vi "Set VI Icon Demo.vi"() -> ()   [LabVIEW 2013]
panel:
  out "Icon File":path
  in  "停止":bool
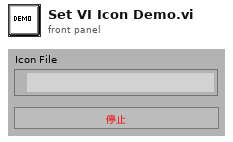
[diagram p1: front panel]
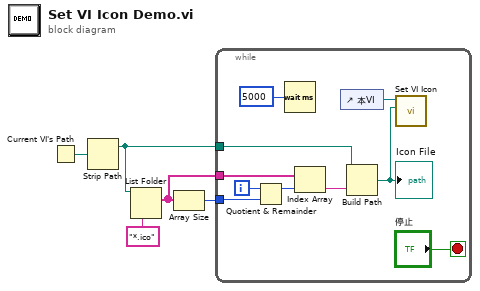
[diagram p0: block diagram]
diagram:
  n1 = Current VI's Path() -> (path=w3:path)
  n2 = Strip Path(path=w3) -> (stripped path=w1:path)  [unwired: 1 out]
  n3 = List Folder(path=w1, pattern="*.ico" ("模式")) -> (filenames=w4:string[])  [unwired: 2 in, 3 out]
  n4 = Array Size(array=w4) -> (size(s)=w5:i32)
  n5 = while {
    tunnel: w5 -> [w12]
    tunnel: w4 -> [w11]
    tunnel: w1 -> [w7]
    i -> [w13]
    stop <- "停止" stop-if-true
    n6 = Quotient & Remainder(x=w13, y=w12) -> (x-y*floor(x/y)=w10:i32)  [unwired: 1 out]
    n7 = Wait (ms)(milliseconds to wait=u32 5000 ("毫秒倍数")) -> ()  [unwired: 1 out]
    n8 = Index Array(array=w11, index=w10) -> (element=w8:string)
    n9 = control-ref of="本VI"() -> (w9:refnum<vi>)
    n10 = Build Path(base path=w7, name or relative path=w8) -> (appended path=w6:path)
    "Icon File" <- w6
    n11 = call "Set VI Icon.vi"("路径"=w6, "VI引用句柄"=w9) -> ()  [unwired: 7 in, 3 out]
  }
